vi "态-路径.vi"(6 "默认值":path, 8 "error in (no error)":errorcluster caption="错误输入（无错误）", 10 "写入":path, 11 "项目开发助手.lvlib:模板-配置文件相关.lvlib:段-.lvclass":refnum<class "段-.lvclass">) -> (0 "error out":errorcluster caption="错误输出", 2 "value":path, 3 "项目开发助手.lvlib:模板-配置文件相关.lvlib:段-.lvclass 2":refnum<class "段-.lvclass">)   [LabVIEW 2017, in "项目开发助手.lvlib" / "模板-配置文件相关.lvlib" / "段-.lvclass"]
uses:
  <vilib>/Utility/config.llb/Not A Config Data Refnum.vi
  <vilib>/Utility/config.llb/Read Key (Path).vi
  <vilib>/Utility/config.llb/Write Key (Path).vi
  <vilib>/Utility/config.llb/NI_LVConfig.lvlib
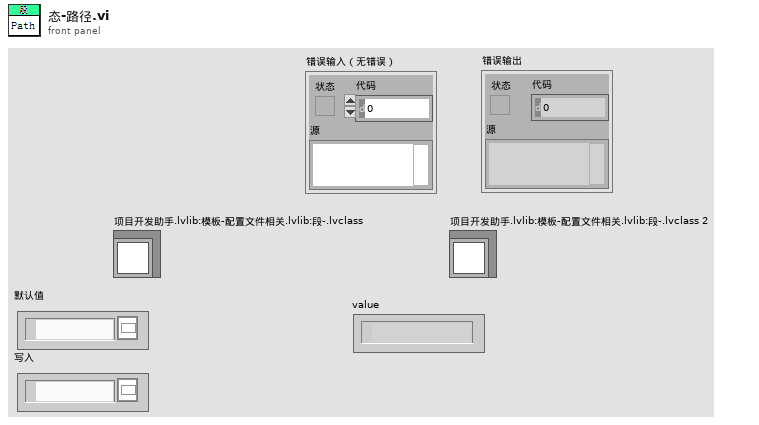
[diagram p1: front panel]
types:
  T1 = typedef "NI_LVConfig.lvlib/Config Data RefNum.ctl" = refnum<k1>
  T2 = typedef "项目开发助手.lvlib/模板-配置文件相关.lvlib/簇-配置文件段键对.ctl" = cluster{"段名":string, "键名":string, "动作":enum16{"读取", "写入"}}
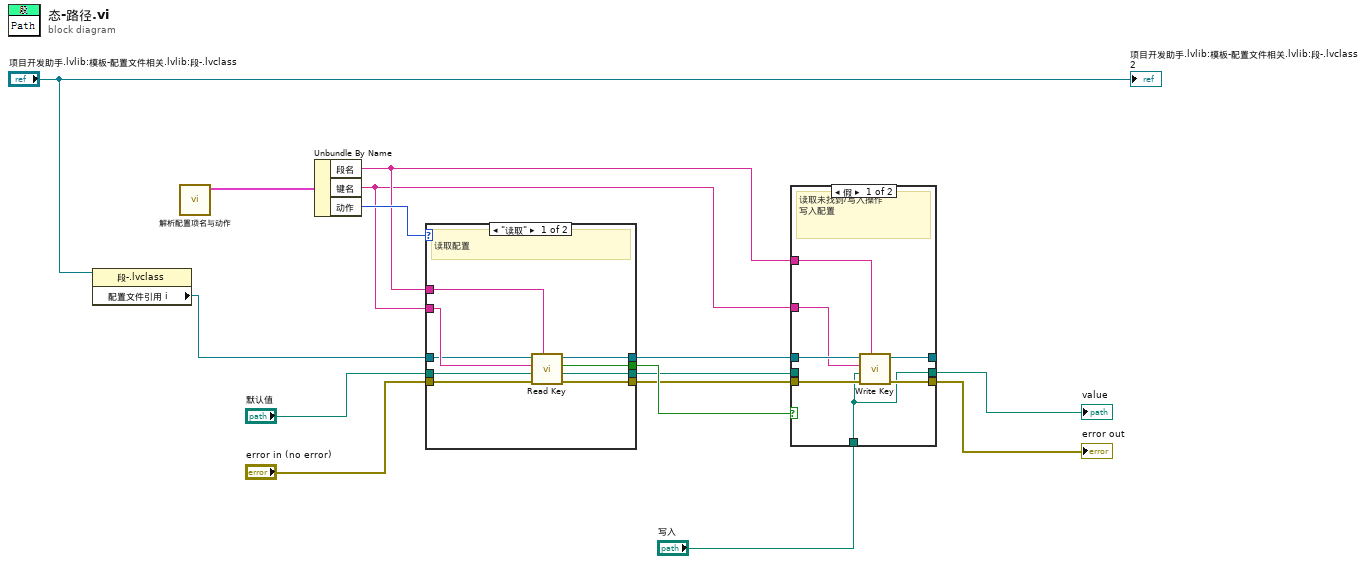
[diagram p0: block diagram]
diagram:
  n1 = property class="段-.lvclass"(reference="项目开发助手.lvlib:模板-配置文件相关.lvlib:段-.lvclass") -> ("配置文件引用 i"=w1:T1)  [unwired: 1 in, 2 out]
  n2 = call "解析配置项名与动作.vi"() -> ("配置项解析"=w3:T2)  [unwired: 10 in, 1 out]
  n3 = Unbundle By Name(w3) -> ("段名"=w9:string, "键名"=w8:string, "动作"=w13:enum16{"读取", "写入"})
  n4 = case shown="\"读取\"" w13 {
    tunnel: w8 -> [w24 _]
    tunnel: w9 -> [w23 _]
    tunnel: w1 -> [w22 w26]
    tunnel: [w21 w26] -> w10
    tunnel: [w20 w25] -> w11
    tunnel: "error in (no error)" -> [w19 w25]
    tunnel: "默认值" -> [w18 _]
    tunnel: [w17 _] -> w5
    tunnel: [w16 _] -> w12
    frame "读取" {
      # "读取配置"
      n5 = call-poly <vilib>:"Read Key.vi"("section"=w23, "error in (no error)"=w19, "default value"=w18, "key"=w24, "refnum"=w22) -> ("error out"=w20:errorcluster, "value"=w17:path, "found?"=w16:bool, "refnum out"=w21:T1)  [unwired: 3 in]
    }
    frame "写入" {
    }
  }
  n6 = case shown="假" w12 {
    tunnel: w11 -> [w29 w35]
    tunnel: w10 -> [w33 w34]
    tunnel: [w32 w34] -> _
    tunnel: w9 -> [w31 _]
    tunnel: w8 -> [w30 _]
    tunnel: "写入" -> [w27 _]
    tunnel: [w28 w35] -> w6
    tunnel: w5 -> [_ w36]
    tunnel: [w27 w36] -> w4
    frame False {
      # "读取未找到/写入操作\n写入配置"
      n7 = call-poly <vilib>:"Write Key.vi"("section"=w31, "error in (no error)"=w29, "value"=w27, "key"=w30, "refnum"=w33) -> ("error out"=w28:errorcluster, "refnum out"=w32:T1)  [unwired: 4 in, 1 out]
    }
    frame True {
    }
  }
  "error out" <- w6
  "value" <- w4
  "项目开发助手.lvlib:模板-配置文件相关.lvlib:段-.lvclass 2" <- "项目开发助手.lvlib:模板-配置文件相关.lvlib:段-.lvclass"
